vi "Test Plot Interpolation Conversion.vi"() -> ()   [LabVIEW 2021, in "Graphs.lvlib"]
uses:
  LabVIEW Plot Interpolation.ctl
  Graphs.lvlib
  <vilib>/measure/NI_MABase.lvlib
panel:
  in  "Plot Interpolation (List)":T1=enum."Line (-)"
  in  "Set Interpolation Style":bool
  out "Plot Interpolation (Property Node)":u8
  out "Waveform Graph":waveform(dbl)(graph)
  # "With checkbox off, change plot interpolation style and run to read PN\n                                                             |\n                                                             |"
  # "<--- Check this box to test List >> PN conversion"
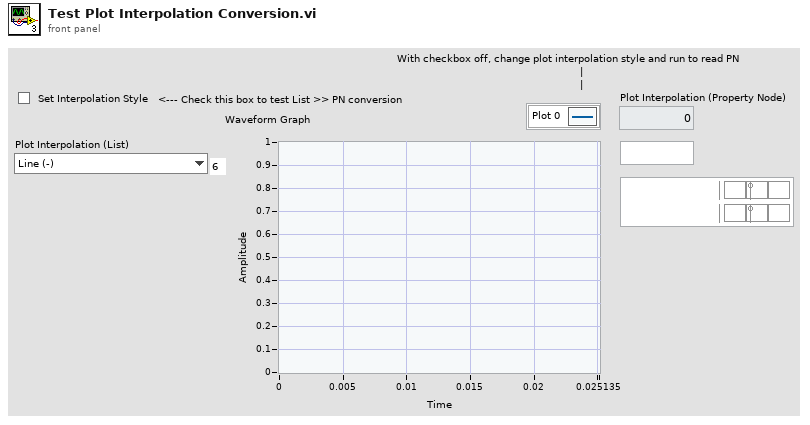
[diagram p1: front panel]
types:
  T1 = typedef "Graphs.lvlib/LabVIEW Plot Interpolation.ctl" = enum16{"Point (.)", "Stepwise Right (--.)", "Line + Point (\\. /)", "Stepwise Left (.--)", "Stepwise Centered (-.-)", "Stepwise Vertical (|.|)", "Line (-)", "Use Previous Plot's Style"}
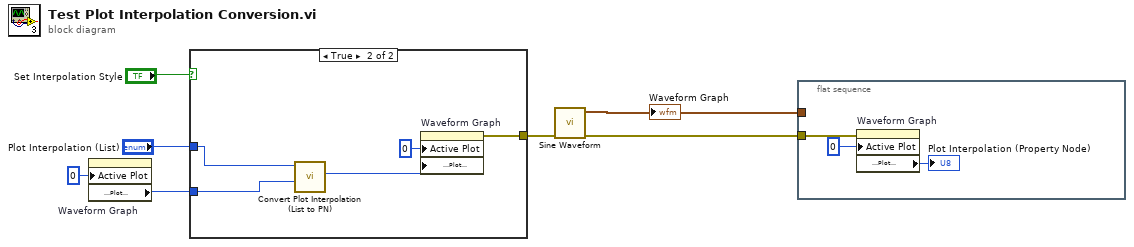
[diagram p0: block diagram]
diagram:
  n1 = property on="Waveform Graph" class="WFGraph (strict)"("Active Plot"=u32 0) -> ("Plot.Plot Interpolation"=w1:u8)  [unwired: 2 in, 2 out]
  n2 = case shown="True" "Set Interpolation Style" {
    tunnel: [_ w11] -> w4
    tunnel: "Plot Interpolation (List)" -> [_ w10]
    tunnel: w1 -> [_ w9]
    frame False {
    }
    frame True {
      n3 = call "Convert Plot Interpolation (List to PN).vi"("Plot Interpolation (PN) in"=w9, "Plot Interpolation (List)"=w10) -> ("Plot.Plot Interpolation (PN)"=w8:u8)  [unwired: 8 in, 1 out]
      n4 = property on="Waveform Graph" class="WFGraph (strict)"("Active Plot"=u32 0, "Plot.Plot Interpolation"=w8) -> (error out=w11:errorcluster)  [unwired: 2 in, 1 out]
    }
  }
  n5 = call <vilib>:"Sine Waveform.vi"("error in (no error)"=w4) -> ("error out"=w7:errorcluster, "signal out"=w6:waveform(dbl))  [unwired: 9 in]
  "Waveform Graph" <- w6
  n6 = flat-sequence {
    tunnel: w7 -> [w15]
    tunnel: w6 -> [_]
    frame #0 {
      n7 = property on="Waveform Graph" class="WFGraph (strict)"(error in=w15, "Active Plot"=u32 0) -> ("Plot.Plot Interpolation"=→"Plot Interpolation (Property Node)":u8)  [unwired: 1 in, 2 out]
    }
  }
